vi "EnFlo_Hub.vi"() -> ()   [LabVIEW 2011]
uses:
  Anemometry Sub Vis/Controls/Launch_controls/Open_Calib.ctl
  Anemometry Sub Vis/Controls/Launch_controls/Open_Meas.ctl
  Anemometry Sub Vis/Controls/Launch_controls/Open_Enter_Temp.ctl
  Anemometry Sub Vis/Controls/Launch_controls/Multi_Run_Prog.ctl
  Anemometry Sub Vis/Controls/Launch_controls/EnFlo_arm.ctl
  Anemometry Sub Vis/Controls/Launch_controls/Fast_FID_Valve.ctl
  Anemometry Sub Vis/Controls/Launch_controls/Disp_Setup.ctl
  Anemometry Sub Vis/Controls/Launch_controls/EnFlo_Tun_Setup.ctl
  Anemometry Sub Vis/Controls/Launch_controls/User_Metadata.ctl
  Anemometry Sub Vis/Controls/Launch_controls/Trav_3D_move.ctl
  Anemometry Sub Vis/Controls/Launch_controls/Trav_Space.ctl
  Anemometry Sub Vis/Controls/Launch_controls/Tunnel_speed.ctl
  Anemometry Sub Vis/Controls/Launch_controls/Client_source_control.ctl
  Anemometry Sub Vis/Controls/Launch_controls/Hydrosonic_Manual.ctl
  Anemometry Sub Vis/Controls/Launch_controls/Preference_Panel.ctl
  Anemometry Sub Vis/Controls/Launch_controls/Hot_wire_Calculator.ctl
  Anemometry Sub Vis/Controls/Launch_controls/RW_X_Parker_Config.ctl
  Anemometry Sub Vis/Controls/Launch_controls/LDA_Alignment.ctl
  Anemometry Sub Vis/Controls/Launch_controls/Named_Serial_Comms.ctl
  Anemometry Sub Vis/Controls/Launch_controls/BSA_data_rates.ctl
  Anemometry Sub Vis/Controls/Launch_controls/Serial_Setup.ctl
  Anemometry Sub Vis/Controls/Launch_controls/Post_Process_icon.ctl
  Anemometry Sub Vis/Controls/Launch_controls/Edit_Ascii_file.ctl
  Anemometry Sub Vis/Controls/Launch_controls/Edit_Raw_DF.ctl
  Anemometry Sub Vis/Controls/Launch_controls/Results_file_plotter.ctl
  Anemometry Sub Vis/Controls/Launch_controls/Serial_Port_Names.ctl
  Anemometry Sub Vis/Controls/Launch_controls/Enter_LDA_Setup.ctl
  Anemometry Sub Vis/Controls/Launch_controls/Paul.ctl
  Anemometry Sub Vis/Controls/Launch_controls/Tom.ctl
  Anemometry Sub Vis/Controls/Launch_controls/Scani_Valve.ctl
  Anemometry Sub Vis/Controls/Launch_controls/Edit_sever_Channel.ctl
  Anemometry Sub Vis/Controls/Launch_controls/Day_file_plotter.ctl
  Anemometry Sub Vis/Controls/Launch_controls/Plot_Sever_Data.ctl
  Anemometry Sub Vis/Controls/Launch_controls/Adam_Table.ctl
  Anemometry Sub Vis/Controls/Launch_controls/Active_Channel_Control.ctl
  Anemometry Sub Vis/Controls/Setup.ctl
  Anemometry Sub Vis/Controls/Post_Process.ctl
  Anemometry Sub Vis/Controls/Preference_Mode.ctl
  Anemometry Sub Vis/Gen Trav/Trav_mode.ctl
  Anemometry Sub Vis/Controls/User_Specific_mode.ctl
  Anemometry Sub Vis/File/Setup_Filetype.ctl
  Anemometry Sub Vis/Calibration/Calib_mode.ctl
  Anemometry Sub Vis/Controls/App_Global.ctl
  Anemometry Sub Vis/Globals/Dynamic_call_global.ph.vi
  Anemometry Sub Vis/Globals/Constants_global.vi
  Anemometry Sub Vis/Globals/Preference_global.vi
  Anemometry Sub Vis/Globals/Meas_global.vi
  <vilib>/Platform/browser.llb/Open URL in Default Browser (string).vi
  Anemometry Sub Vis/Globals/Trav_pos_global.vi
  Anemometry Sub Vis/Globals/Qnet_Globals.vi
  Anemometry Sub Vis/Acquisition/PWA/PWAtasksGLOBAL.vi
  Anemometry Sub Vis/Utilities/Email_transfer_global.vi
panel:
  out "List of ADAM channels to view":string[](array[string])
  out "List of ADAM control channels":string[](array[string])
  out "Analogue Dev Name":string="Dev2"
  out "Numeric":i32
  out "Rig Name":string="EnFlo Tunnel"
  out "All Users":path=path "/System Folder/Preferences/LabVIEW (EnFlo specific)/Meas Setups"
  out "Dummy Measurement":bool
  out "Ready to take data?":T1
  out "Local Site Root":path=path "/Lacie_20/paulhayden/Qnet/qnet"
  in  "stop":bool
  in  "Tab Control":T2(tab)
  in  "Tunnel Speed Control":T3
  in  "Traverse Space":T4
  in  "Trav 3D Move":T5 caption="3D Traverse Move"
  in  "User Metadata":T6
  in  "Multi Run Prog":T7
  in  "Enter Temp_Press":T8
  in  "Measurement Prog":T9 caption="Measurement"
  in  "Calibration Prog":T10 caption="Calibration"
  in  "Scani Valve":T11
  in  "LDA Alignment":T12
  in  "Hydrosonic Control":T13
  in  "Fast FID Valve":T14
  in  "Source Control":T15
  in  "Gas Release Setup":T16
  in  "EnFlo Tunnel Setup":T17
  in  "Heater Setup":bool caption="Inlet heater File"
  in  "EnFlo Arm":T18
  in  "Rig_Control":cluster{"Ch Name":string, "Boolean":bool}[](array[cluster])
  in  "ADAM Channels Control":T19 caption="Change Active Channels"
  in  "ADAM Scan Table":T20 caption="Run ADAM Scan Table"
  in  "Edit Server Channel":T21
  in  "Plot Server Channels":T22 caption="Plot Server Data"
  in  "Day Files Plotter":T23 caption="Plot Data From File"
  out "Current Values":cluster{"Ch Name":string, "Numeric":dbl}[](array[cluster])
  in  "Results File Plotter":T24
  in  "Edit Raw Data Files":T25
  in  "Edit ASCII File":T26
  in  "Post Process Raw Data":T27
  in  "LDA Setup":T28
  in  "Port Names":T29
  in  "Serial Setup":T30
  in  "LDA Data Rate":T31
  in  "Named Serial Comms":T32
  in  "RW Trav Setup":T33
  in  "Hot Wire Calc":T34
  in  "Preference Panel":T35
  in  "Tom Lawton t.lawton@surrey.ac.uk":T36 caption="For hardware support"
  in  "Paul Hayden p.hayden@surrey.ac.uk":T37 caption="For software support"
  in  "Online Manual":bool
  out "VI Name":string
  out "Iterations":i32
  # "Or give us a call on Tel: 01483 689545"
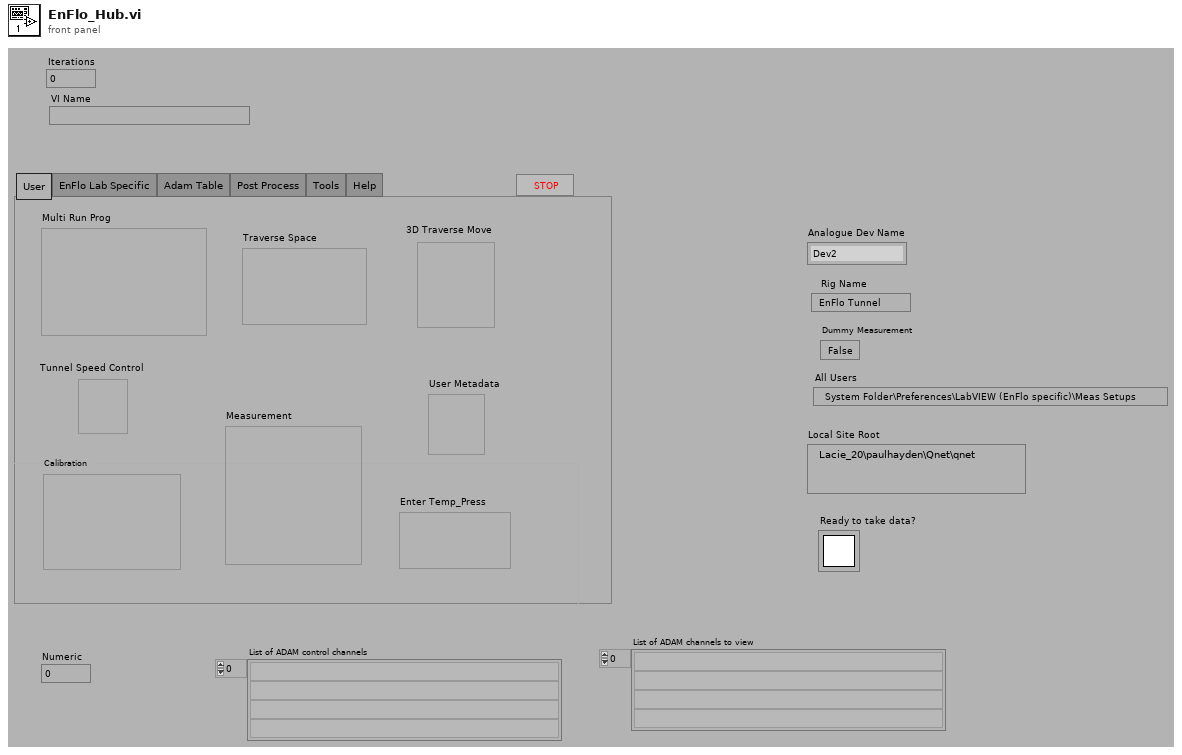
[diagram p1: front panel]
types:
  T1 = typedef "Rendezvous RefNum" = refnum<k1>
  T2 = enum32{"User", "EnFlo Lab Specific", "Adam Table", "Post Process", "Tools", "Help"}
  T3 = typedef "Tunnel_speed.ctl" = bool
  T4 = typedef "Trav_Space.ctl" = bool
  T5 = typedef "Trav_3D_move.ctl" = bool
  T6 = typedef "User_Metadata.ctl" = bool
  T7 = typedef "Multi_Run_Prog.ctl" = bool
  T8 = typedef "Open_Enter_Temp.ctl" = bool
  T9 = typedef "Open_Meas.ctl" = bool
  T10 = typedef "Open_Calib.ctl" = bool
  T11 = typedef "Scani_Valve.ctl" = bool
  T12 = typedef "LDA_Alignment.ctl" = bool
  T13 = typedef "Hydrosonic_Manual.ctl" = bool
  T14 = typedef "Fast_FID_Valve.ctl" = bool
  T15 = typedef "Client_source_control.ctl" = bool
  T16 = typedef "Disp_Setup.ctl" = bool
  T17 = typedef "EnFlo_Tun_Setup.ctl" = bool
  T18 = typedef "EnFlo_arm.ctl" = bool
  T19 = typedef "Active_Channel_Control.ctl" = bool
  T20 = typedef "Adam_Table.ctl" = bool
  T21 = typedef "Edit_sever_Channel.ctl" = bool
  T22 = typedef "Plot_Sever_Data.ctl" = bool
  T23 = typedef "Day_file_plotter.ctl" = bool
  T24 = typedef "Results_file_plotter.ctl" = bool
  T25 = typedef "Edit_Raw_DF.ctl" = bool
  T26 = typedef "Edit_Ascii_file.ctl" = bool
  T27 = typedef "Post_Process_icon.ctl" = bool
  T28 = typedef "Enter_LDA_Setup.ctl" = bool
  T29 = typedef "Serial_Port_Names.ctl" = bool
  T30 = typedef "Serial_Setup.ctl" = bool
  T31 = typedef "BSA_data_rates.ctl" = bool
  T32 = typedef "Named_Serial_Comms.ctl" = bool
  T33 = typedef "RW_X_Parker_Config.ctl" = bool
  T34 = typedef "Hot_wire_Calculator.ctl" = bool
  T35 = typedef "Preference_Panel.ctl" = bool
  T36 = typedef "Tom.ctl" = bool
  T37 = typedef "Paul.ctl" = bool
  T38 = typedef "Post_Process.ctl" = enum16{"Take New Data", "Post Process Raw Data File"}
  T39 = typedef "Setup.ctl" = enum16{"Run Program", "Show Setup", "Save Current Setup", "Setup Front Panel"}
  T40 = enum16{"Get Channel Names", "Get Current Value", "Update Channel Value", "Update Channel Description"}
  T41 = typedef "Preference_Mode.ctl" = enum16{"Load Preferences from file", "Save Preferences to file", "Load, Edit then Save"}
  T42 = typedef "User_Specific_mode.ctl" = enum16{"Check VI only", "Run VI"}
  T43 = typedef "Trav_mode.ctl" = enum16{"Move traverse", "Read traverse position", "Teach Position"}
  T44 = typedef "Setup_Filetype.ctl" = enum16{"Measurement Setups", "Calibration Setups", "General", "Results File Plotter Setups", "Speed Calib Tweaks"}
  T45 = enum16{"Load Command File", "Save Command File", "Check Multi Run Prog", "Check Multi Run Prog With Live Moves", "Run Multi Run Prog"}
  T46 = typedef "Calib_mode.ctl" = enum16{"Show Setup", "Take a New Calibration Point", "Refit Curve", "Setup Front Panel"}
  T47 = typedef "Tunnel_Coordinates.ctl" = enum16{"Work in Tunnel Coordinates", "Work in Model Coordinates"}
  T48 = typedef "App_Global.ctl" = enum16{"Read Global", "Write to Global", "Initialise Array"}
  T49 = typedef "App_Ref_Cluster.ctl" = cluster{"Server IP & Port No":string, "Application reference":refnum<vi>}
  T50 = typedef "Ch_description_ADAM.ctl" = cluster{"Ch Name":string, "Type":T51, "Function":T52, "Ch State":T53, "Calibration type":T54, "A":dbl, "B":dbl, "C":dbl, "D":dbl, "Comments":string, "Address":T55, "String":string, "Duty":u16}
  T51 = typedef "Module_type_ADAM.ctl" = string
  T52 = typedef "Function_ADAM.ctl" = enum16{"Analogue Input", "Digital Input", "Event counter", "Event rate", "Analogue Output", "Digital Output", "Relay Output"}
  T53 = typedef "Channel_State.ctl" = enum16{"On", "Off", "Always On", "Always Off"}
  T54 = typedef "Calib_type_ADAM.ctl" = enum16{"Raw", "Bx + A", "Cx^2 + Bx + A", "Dx^3 + Cx^2 + Bx + A", "In Band", "Hi-Tec Q", "Hi-Tec M_dot", "Text"}
  T55 = typedef "Address.ctl" = cluster{"Main":i32, "Ch.":i32, "Sub":i32, "Port Name":string}
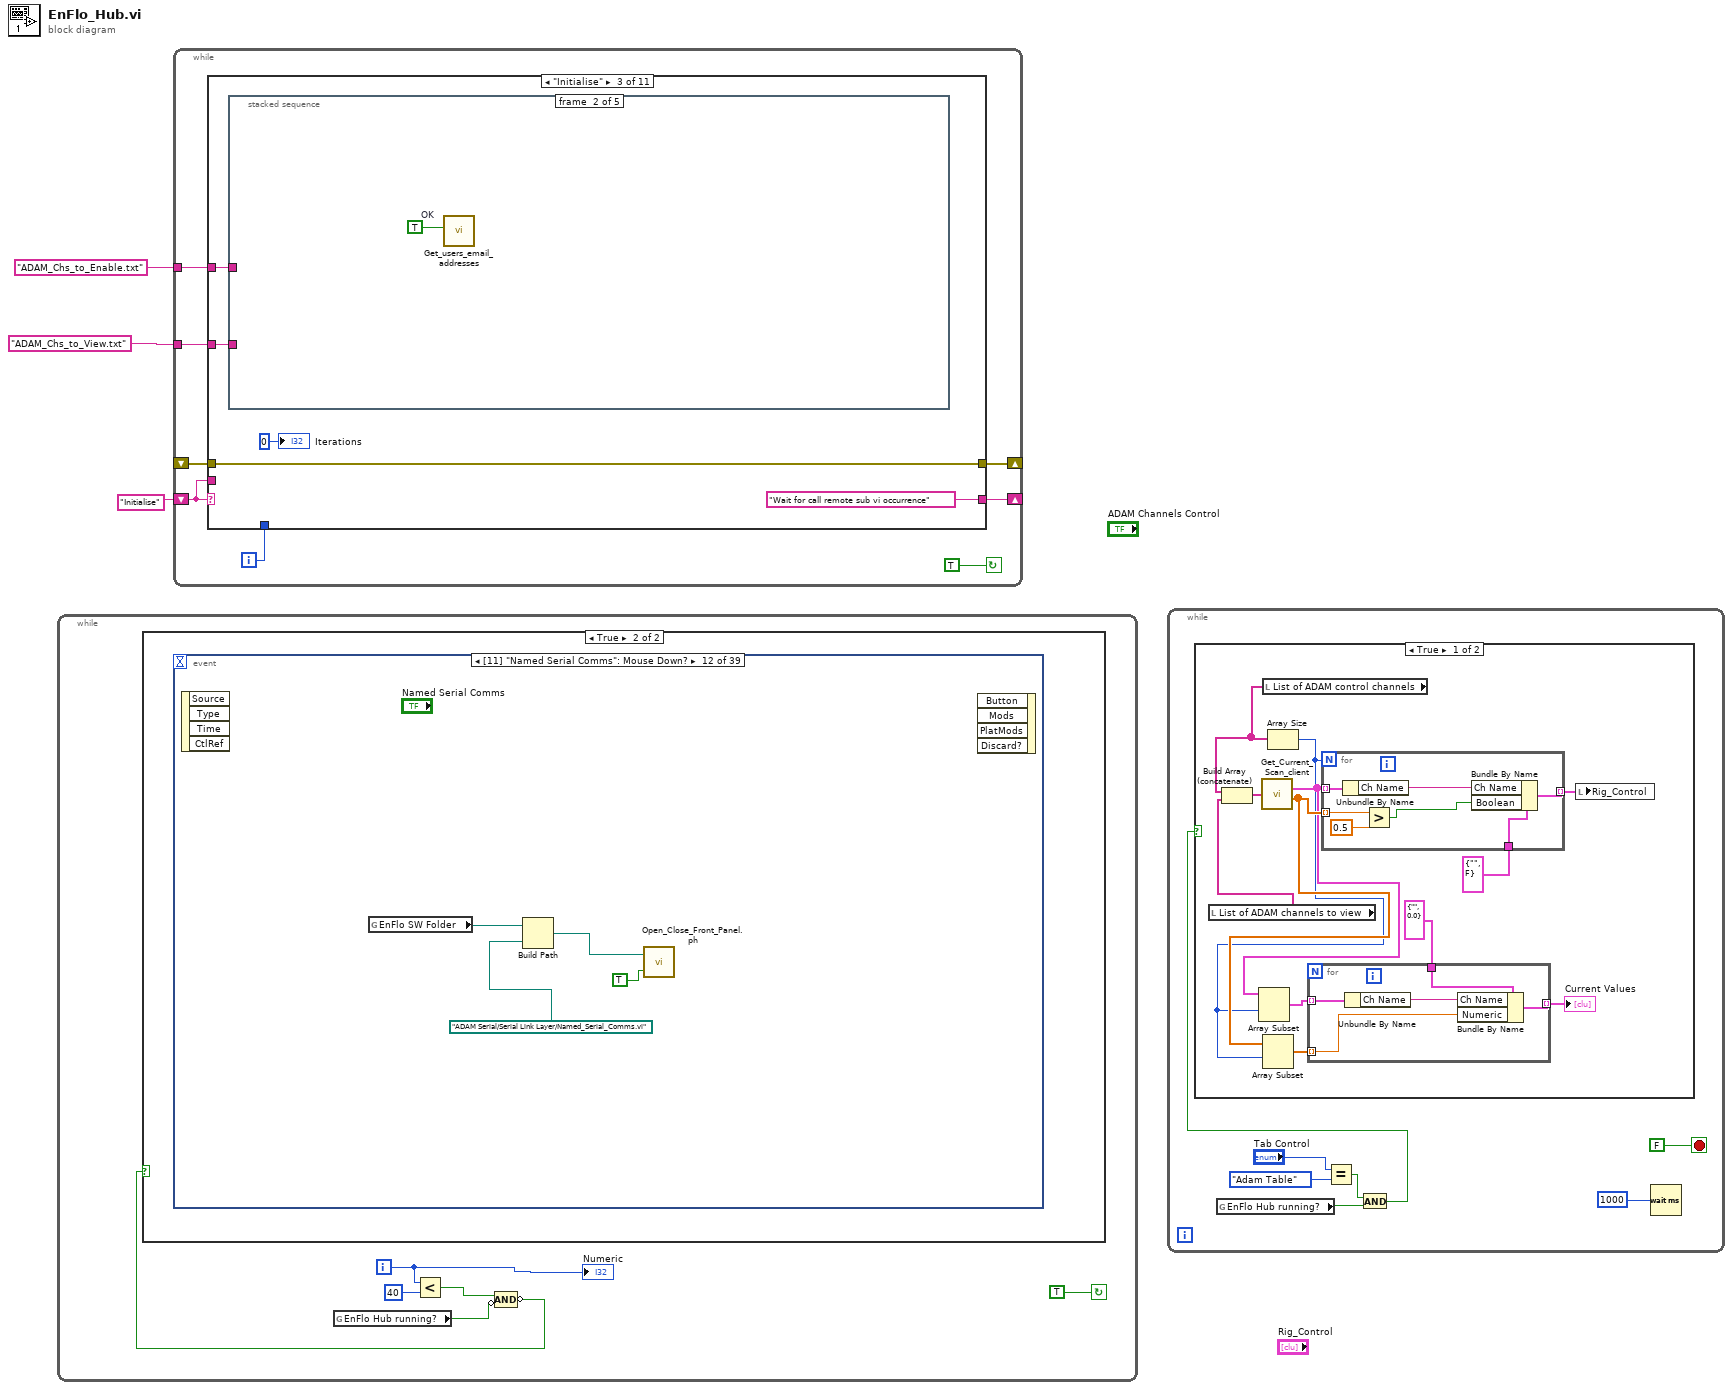
[diagram p0: block diagram]
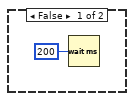
[diagram p3: hidden frame]
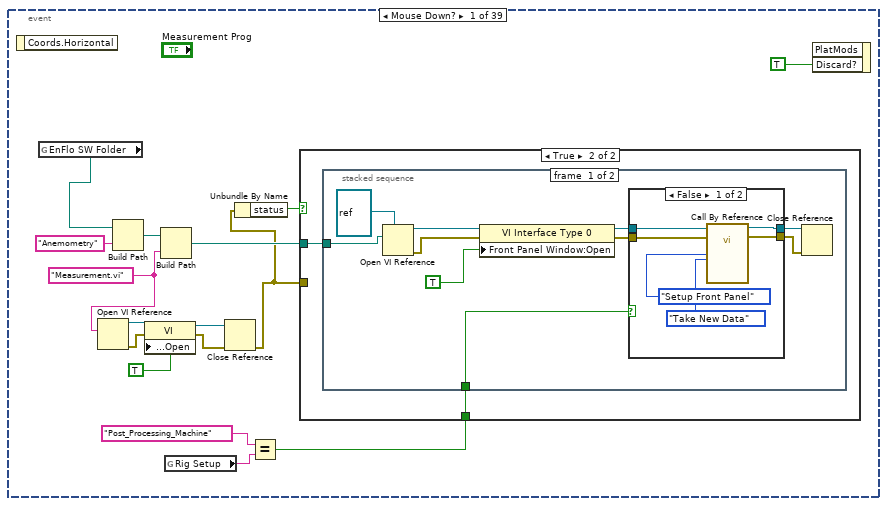
[diagram p4: hidden frame]
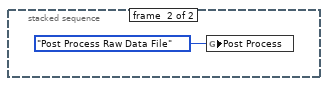
[diagram p7: hidden frame]
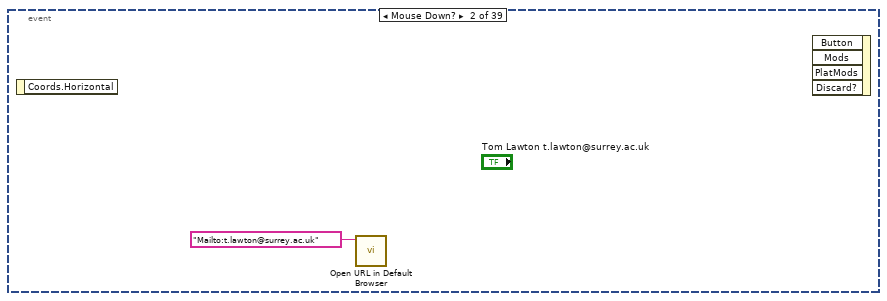
[diagram p8: hidden frame]
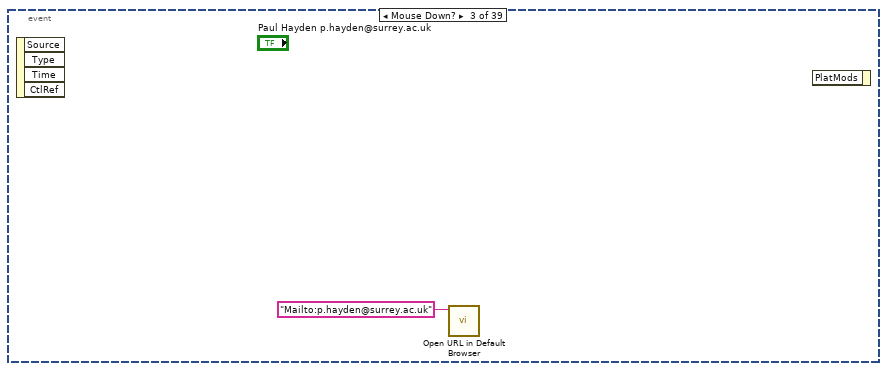
[diagram p9: hidden frame]
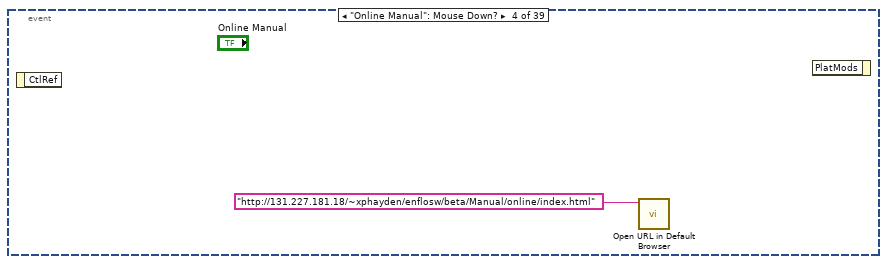
[diagram p10: hidden frame]
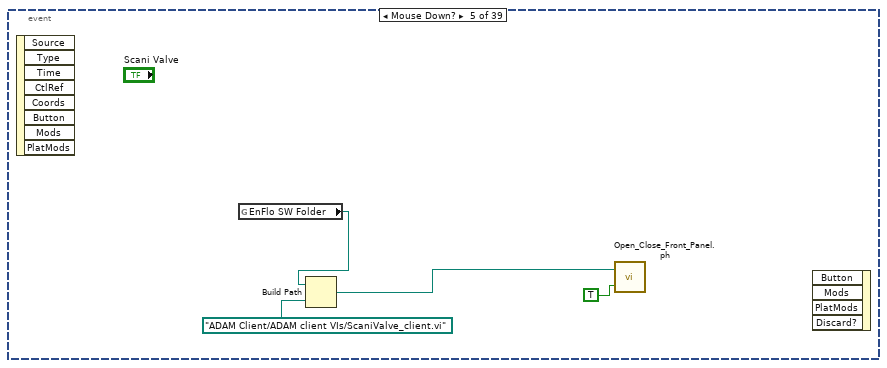
[diagram p11: hidden frame]
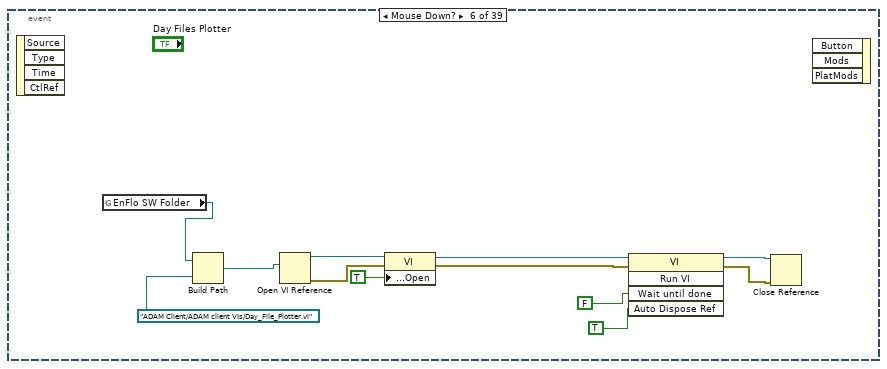
[diagram p12: hidden frame]
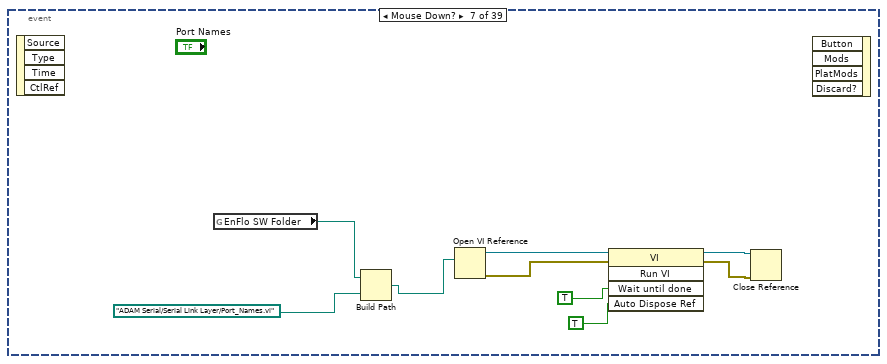
[diagram p13: hidden frame]
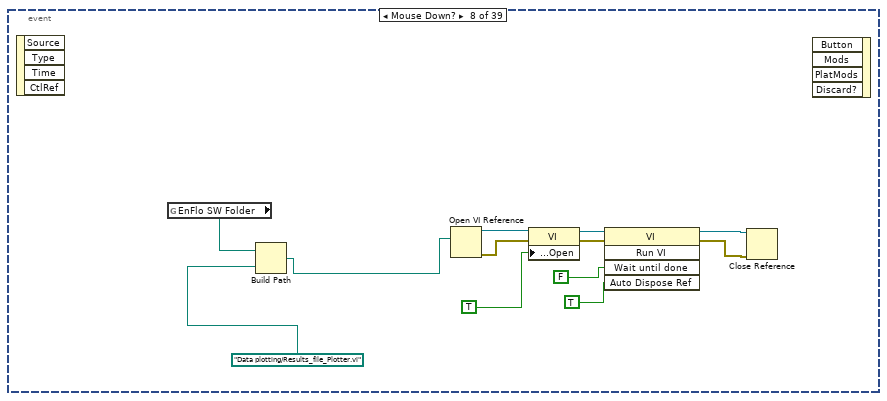
[diagram p14: hidden frame]
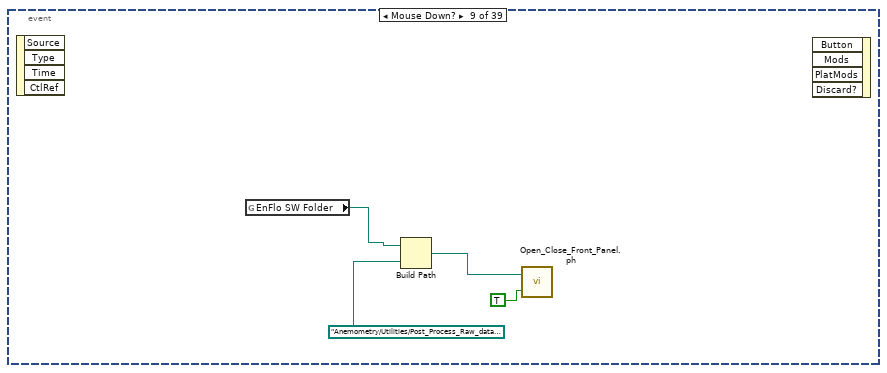
[diagram p15: hidden frame]
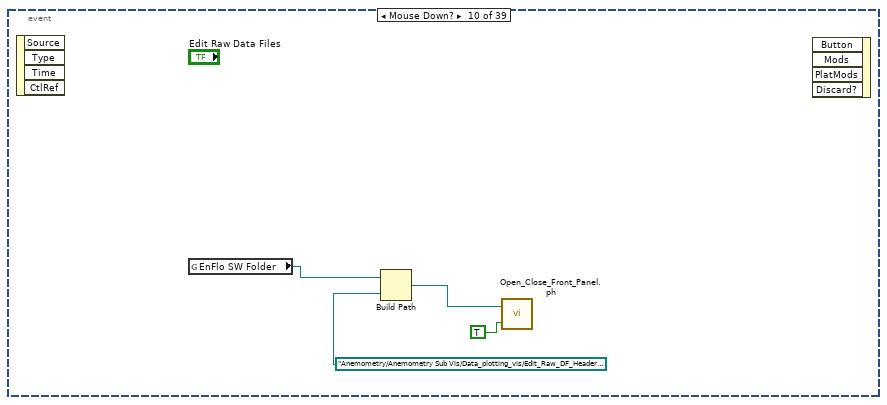
[diagram p16: hidden frame]
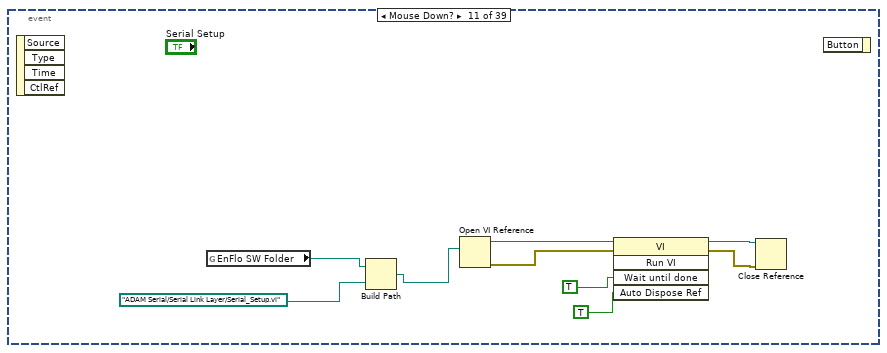
[diagram p17: hidden frame]
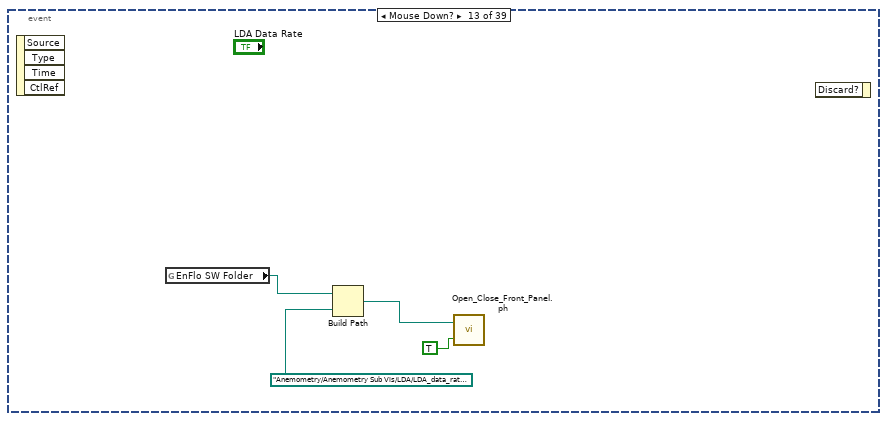
[diagram p18: hidden frame]
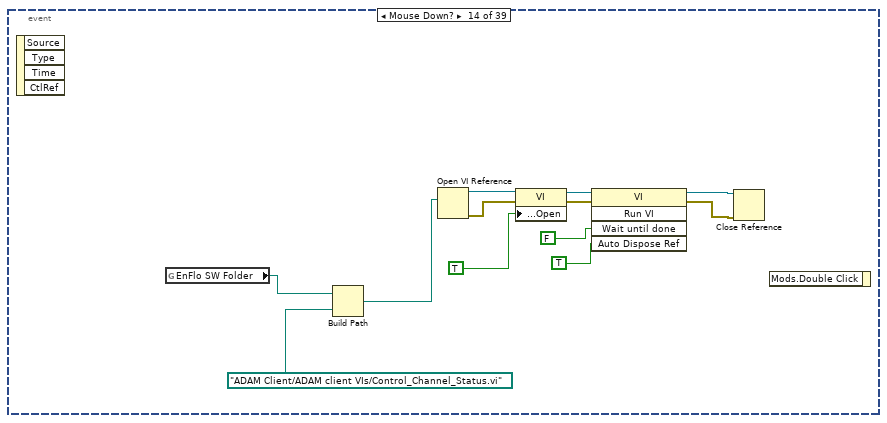
[diagram p19: hidden frame]
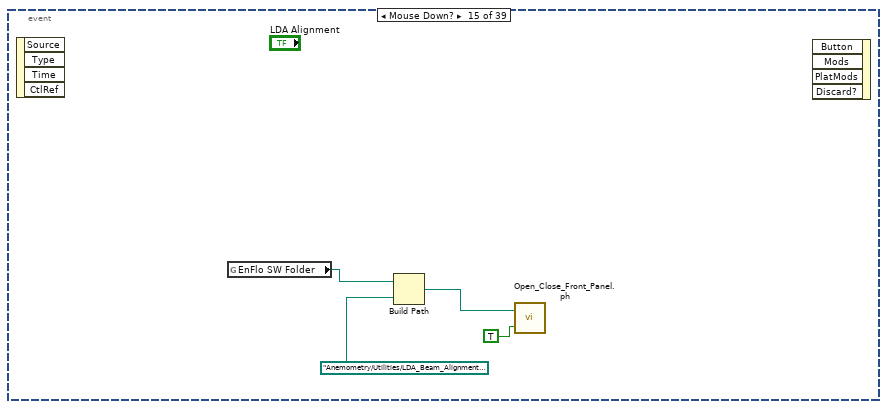
[diagram p20: hidden frame]
diagram:
  n1 = while {
    i -> [w8]
    stop <- TRUE continue-if-true
    n2 = global read "Dynamic_call_global.ph.vi" "EnFlo Hub running?"() -> (w6:bool)
    n3 = Less?(x=w8, y=40) -> (x < y?=w5:bool)
    n4 = Compound Arithmetic op=AND(w5, invert w6) -> (invert w4:bool)
    n5 = case shown="True" w4 {
      frame False {
        n6 = Wait (ms)(milliseconds to wait=u32 200) -> ()  [unwired: 1 out]
      }
      frame True {
        n7 = event shown="[11] \"Named Serial Comms\": Mouse Down?" {
          selector: _ -> [_ _ _ _ _ _ _ _ _ _ _ _ _ _ _ _ _ _ _ _ _ _ _ _ _ _ _ _ _ _ _ _ _ _ _ _ _ _ _]
          dyn-events: _ -> [_ _ _ _ _ _ _ _ _ _ _ _ _ _ _ _ _ _ _ _ _ _ _ _ _ _ _ _ _ _ _ _ _ _ _ _ _ _ _]
          timeout: _ -> [_ _ _ _ _ _ _ _ _ _ _ _ _ _ _ _ _ _ _ _ _ _ _ _ _ _ _ _ _ _ _ _ _ _ _ _ _ _ _]
          event Mouse Down? {
            w19 = "Measurement.vi" ("name or relative path")
            n8 = event-data() -> ()  [unwired: 2 out]
            n9 = global read "Constants_global.vi" "EnFlo SW Folder"() -> (w22:path)
            n10 = Open VI Reference(vi path=w19) -> (vi reference=w18:refnum<vi>, error out=w17:errorcluster)  [unwired: 1 in, 4 out]
            n11 = Build Path(base path=w22, name or relative path="Anemometry") -> (appended path=w25:path)
            n12 = property class="VI"(reference=w18, error in=w17, "Front Panel Window:Open"=TRUE) -> (reference out=w15:refnum<vi>, error out=w16:errorcluster)
            n13 = Build Path(base path=w25, name or relative path=w19) -> (appended path=w23:path)
            n14 = global read "Preference_global.vi" "Rig Setup"() -> (w13:string)
            n15 = Close Reference(reference=w15, error in (no error)=w16) -> (error out=w14:errorcluster)
            n16 = Unbundle By Name(w14) -> ("status"=w24:bool)
            n17 = Equal?(x="Post_Processing_Machine" ("Rig Setup"), y=w13) -> (x = y?=w11:bool)
            n18 = case shown="True" w24 {
              tunnel: w23 -> [_ w28]
              tunnel: w14 -> [_ _]
              tunnel: w11 -> [_ w27]
              frame False {
              }
              frame True {
                n19 = stacked-sequence {
                  tunnel: w28 -> [w38 _]
                  tunnel: w27 -> [w29 _]
                  frame #0 {
                    n20 = Open VI Reference(type specifier VI Refnum (for type only)=refnum<vi> refnum, vi path=w38) -> (vi reference=w36:refnum<vi>, error out=w35:errorcluster)  [unwired: 1 in, 3 out]
                    n21 = property class="VI Interface Type 0"(reference=w36, error in=w35, "Front Panel Window:Open"=TRUE) -> (reference out=w31:refnum<vi>, error out=w30:errorcluster)
                    n22 = case shown="False" w29 {
                      tunnel: [w44 w46] -> w34
                      tunnel: [w43 w45] -> w33
                      tunnel: w31 -> [w42 w46]
                      tunnel: w30 -> [w41 w45]
                      frame False {
                        n23 = call-by-ref "?"(reference=w42, error in=w41, "setup"=Setup."Setup Front Panel", "Post Process"=Post_Process."Take New Data") -> (reference out=w44:refnum<vi>, error out=w43:errorcluster)  [unwired: 16 in, 2 out]
                      }
                      frame True {
                      }
                    }
                    n24 = Close Reference(reference=w34, error in (no error)=w33) -> ()  [unwired: 1 out]
                  }
                  frame #1 {
                    n25 = global write "Meas_global.vi" "Post Process"(Post_Process."Post Process Raw Data File" ("Post Process")) -> ()
                  }
                }
              }
            }
            n26 = event-data("Discard?"=TRUE) -> ()  [unwired: 1 in, 2 out]
          }
          event Mouse Down? {
            n27 = event-data() -> ()  [unwired: 2 out]
            n28 = call-poly <vilib>:"Open URL in Default Browser.vi"("URL"="Mailto:t.lawton@surrey.ac.uk") -> ()  [unwired: 1 in, 6 out]
            n29 = event-data() -> ()  [unwired: 1 in, 5 out]
          }
          event Mouse Down? {
            n30 = event-data() -> ()  [unwired: 5 out]
            n31 = call-poly <vilib>:"Open URL in Default Browser.vi"("URL"="Mailto:p.hayden@surrey.ac.uk") -> ()  [unwired: 1 in, 6 out]
            n32 = event-data() -> ()  [unwired: 1 in, 2 out]
          }
          event "Online Manual": Mouse Down? {
            n33 = event-data() -> ()  [unwired: 2 out]
            n34 = call-poly <vilib>:"Open URL in Default Browser.vi"("URL"="http://131.227.181.18/~xphayden/enflosw/beta/Manual/online/index.html") -> ()  [unwired: 1 in, 6 out]
            n35 = event-data() -> ()  [unwired: 1 in, 2 out]
          }
          event Mouse Down? {
            n36 = event-data() -> ()  [unwired: 9 out]
            n37 = global read "Constants_global.vi" "EnFlo SW Folder"() -> (w51:path)
            n38 = Build Path(base path=w51, name or relative path=path "ADAM Client/ADAM client VIs/ScaniValve_client.vi") -> (appended path=w54:path)
            n39 = call "Open_Close_Front_Panel.ph.vi"("Front Panel Window:Open"=TRUE, "VI path"=w54) -> ()  [unwired: 2 out]
            n40 = event-data() -> ()  [unwired: 1 in, 5 out]
          }
          event Mouse Down? {
            n41 = event-data() -> ()  [unwired: 5 out]
            n42 = global read "Constants_global.vi" "EnFlo SW Folder"() -> (w55:path)
            n43 = Build Path(base path=w55, name or relative path=path "ADAM Client/ADAM client VIs/Day_File_Plotter.vi") -> (appended path=w61:path)
            n44 = Open VI Reference(vi path=w61) -> (vi reference=w62:refnum<vi>, error out=w64:errorcluster)  [unwired: 2 in, 3 out]
            n45 = property class="VI"(reference=w62, error in=w64, "Front Panel Window:Open"=TRUE) -> (reference out=w66:refnum<vi>, error out=w65:errorcluster)
            n46 = invoke class="VI" method="Run VI"(reference=w66, error in=w65, "Wait until done"=FALSE, "Auto Dispose Ref"=TRUE) -> (reference out=w57:refnum<vi>, error out=w58:errorcluster)  [unwired: 1 in, 3 out]
            n47 = Close Reference(reference=w57, error in (no error)=w58) -> ()  [unwired: 1 out]
            n48 = event-data() -> ()  [unwired: 1 in, 4 out]
          }
          event Mouse Down? {
            n49 = event-data() -> ()  [unwired: 5 out]
            n50 = global read "Constants_global.vi" "EnFlo SW Folder"() -> (w67:path)
            n51 = Build Path(base path=w67, name or relative path=path "ADAM Serial/Serial Link Layer/Port_Names.vi") -> (appended path=w69:path)
            n52 = Open VI Reference(vi path=w69) -> (vi reference=w74:refnum<vi>, error out=w75:errorcluster)  [unwired: 1 in, 4 out]
            n53 = invoke class="VI" method="Run VI"(reference=w74, error in=w75, "Wait until done"=TRUE, "Auto Dispose Ref"=TRUE) -> (reference out=w70:refnum<vi>, error out=w71:errorcluster)  [unwired: 1 in, 3 out]
            n54 = Close Reference(reference=w70, error in (no error)=w71) -> ()  [unwired: 1 out]
            n55 = event-data() -> ()  [unwired: 1 in, 5 out]
          }
          event Mouse Down? {
            n56 = event-data() -> ()  [unwired: 5 out]
            n57 = global read "Constants_global.vi" "EnFlo SW Folder"() -> (w76:path)
            n58 = Build Path(base path=w76, name or relative path=path "Data plotting/Results_file_Plotter.vi") -> (appended path=w79:path)
            n59 = Open VI Reference(vi path=w79) -> (vi reference=w81:refnum<vi>, error out=w78:errorcluster)  [unwired: 1 in, 4 out]
            n60 = property class="VI"(reference=w81, error in=w78, "Front Panel Window:Open"=TRUE) -> (reference out=w82:refnum<vi>, error out=w83:errorcluster)
            n61 = invoke class="VI" method="Run VI"(reference=w82, error in=w83, "Wait until done"=FALSE, "Auto Dispose Ref"=TRUE) -> (reference out=w84:refnum<vi>, error out=w85:errorcluster)  [unwired: 1 in, 3 out]
            n62 = Close Reference(reference=w84, error in (no error)=w85) -> ()  [unwired: 1 out]
            n63 = event-data() -> ()  [unwired: 1 in, 5 out]
          }
          event Mouse Down? {
            n64 = event-data() -> ()  [unwired: 5 out]
            n65 = global read "Constants_global.vi" "EnFlo SW Folder"() -> (w88:path)
            n66 = Build Path(base path=w88, name or relative path=path "Anemometry/Utilities/Post_Process_Raw_data.vi") -> (appended path=w90:path)
            n67 = call "Open_Close_Front_Panel.ph.vi"("Front Panel Window:Open"=TRUE, "VI path"=w90) -> ()  [unwired: 2 out]
            n68 = event-data() -> ()  [unwired: 1 in, 5 out]
          }
          event Mouse Down? {
            n69 = event-data() -> ()  [unwired: 5 out]
            n70 = global read "Constants_global.vi" "EnFlo SW Folder"() -> (w92:path)
            n71 = Build Path(base path=w92, name or relative path=path "Anemometry/Anemometry Sub Vis/Data_plotting_vis/Edit_Raw_DF_Header.vi") -> (appended path=w94:path)
            n72 = call "Open_Close_Front_Panel.ph.vi"("Front Panel Window:Open"=TRUE, "VI path"=w94) -> ()  [unwired: 2 out]
            n73 = event-data() -> ()  [unwired: 1 in, 5 out]
          }
          event Mouse Down? {
            n74 = event-data() -> ()  [unwired: 5 out]
            n75 = global read "Constants_global.vi" "EnFlo SW Folder"() -> (w96:path)
            n76 = Build Path(base path=w96, name or relative path=path "ADAM Serial/Serial Link Layer/Serial_Setup.vi") -> (appended path=w98:path)
            n77 = Open VI Reference(vi path=w98) -> (vi reference=w103:refnum<vi>, error out=w104:errorcluster)  [unwired: 1 in, 4 out]
            n78 = invoke class="VI" method="Run VI"(reference=w103, error in=w104, "Wait until done"=TRUE, "Auto Dispose Ref"=TRUE) -> (reference out=w99:refnum<vi>, error out=w100:errorcluster)  [unwired: 1 in, 3 out]
            n79 = Close Reference(reference=w99, error in (no error)=w100) -> ()  [unwired: 1 out]
            n80 = event-data() -> ()  [unwired: 1 in, 2 out]
          }
          event Mouse Down? {
            n81 = event-data() -> ()  [unwired: 5 out]
            n82 = global read "Constants_global.vi" "EnFlo SW Folder"() -> (w106:path)
            n83 = Build Path(base path=w106, name or relative path=path "ADAM Serial/Serial Link Layer/Named_Serial_Comms.vi") -> (appended path=w108:path)
            n84 = call "Open_Close_Front_Panel.ph.vi"("Front Panel Window:Open"=TRUE, "VI path"=w108) -> ()  [unwired: 2 out]
            n85 = event-data() -> ()  [unwired: 1 in, 5 out]
          }
          event Mouse Down? {
            n86 = event-data() -> ()  [unwired: 5 out]
            n87 = global read "Constants_global.vi" "EnFlo SW Folder"() -> (w109:path)
            n88 = Build Path(base path=w109, name or relative path=path "Anemometry/Anemometry Sub Vis/LDA/LDA_data_rate.vi") -> (appended path=w111:path)
            n89 = call "Open_Close_Front_Panel.ph.vi"("Front Panel Window:Open"=TRUE, "VI path"=w111) -> ()  [unwired: 2 out]
            n90 = event-data() -> ()  [unwired: 1 in, 2 out]
          }
          event Mouse Down? {
            n91 = event-data() -> ()  [unwired: 5 out]
            n92 = global read "Constants_global.vi" "EnFlo SW Folder"() -> (w123:path)
            n93 = Build Path(base path=w123, name or relative path=path "ADAM Client/ADAM client VIs/Control_Channel_Status.vi") -> (appended path=w113:path)
            n94 = Open VI Reference(vi path=w113) -> (vi reference=w116:refnum<vi>, error out=w114:errorcluster)  [unwired: 1 in, 4 out]
            n95 = property class="VI"(reference=w116, error in=w114, "Front Panel Window:Open"=TRUE) -> (reference out=w117:refnum<vi>, error out=w118:errorcluster)
            n96 = invoke class="VI" method="Run VI"(reference=w117, error in=w118, "Wait until done"=FALSE, "Auto Dispose Ref"=TRUE) -> (reference out=w119:refnum<vi>, error out=w120:errorcluster)  [unwired: 1 in, 3 out]
            n97 = Close Reference(reference=w119, error in (no error)=w120) -> ()  [unwired: 1 out]
            n98 = event-data() -> ()  [unwired: 1 in, 2 out]
          }
          event Mouse Down? {
            n99 = event-data() -> ()  [unwired: 5 out]
            n100 = global read "Constants_global.vi" "EnFlo SW Folder"() -> (w125:path)
            n101 = Build Path(base path=w125, name or relative path=path "Anemometry/Utilities/LDA_Beam_Alignment.vi") -> (appended path=w127:path)
            n102 = call "Open_Close_Front_Panel.ph.vi"("Front Panel Window:Open"=TRUE, "VI path"=w127) -> ()  [unwired: 2 out]
            n103 = event-data() -> ()  [unwired: 1 in, 5 out]
          }
          event Mouse Down? {
            w130 = FALSE  # Wait until done
            n104 = event-data() -> ()  [unwired: 5 out]
            n105 = call "Run_Enter_Temp.vi"("Wait until done"=w130) -> ()  [unwired: 1 out]
            n106 = event-data("Discard?"=TRUE) -> ()  [unwired: 1 in, 4 out]
          }
          event Mouse Down? {
            n107 = event-data() -> ()  [unwired: 5 out]
            n108 = global read "Constants_global.vi" "EnFlo SW Folder"() -> (w131:path)
            n109 = Build Path(base path=w131, name or relative path=path "Anemometry/Utilities/Edit_ASCI_file.vi") -> (appended path=w134:path)
            n110 = call "Open_Close_Front_Panel.ph.vi"("Front Panel Window:Open"=TRUE, "VI path"=w134) -> ()  [unwired: 2 out]
            n111 = event-data() -> ()  [unwired: 1 in, 5 out]
          }
          event "Heater Setup": Mouse Down? {
            n112 = event-data() -> ()  [unwired: 5 out]
            n113 = global read "Constants_global.vi" "EnFlo SW Folder"() -> (w135:path)
            n114 = Build Path(base path=w135, name or relative path=path "Anemometry/Utilities/Create_Heater_Setpoints_File.vi") -> (appended path=w138:path)
            n115 = call "Open_Close_Front_Panel.ph.vi"("Front Panel Window:Open"=TRUE, "VI path"=w138) -> ()  [unwired: 2 out]
            n116 = event-data() -> ()  [unwired: 1 in, 5 out]
          }
          event Mouse Down? {
            n117 = event-data() -> ()  [unwired: 5 out]
            n118 = global read "Constants_global.vi" "EnFlo SW Folder"() -> (w139:path)
            n119 = Build Path(base path=w139, name or relative path=path "ADAM Client/Sub VIs/Gas_Release_Control.vi") -> (appended path=w142:path)
            n120 = call "Open_Close_Front_Panel.ph.vi"("Front Panel Window:Open"=TRUE, "VI path"=w142) -> ()  [unwired: 2 out]
            n121 = event-data() -> ()  [unwired: 1 in, 5 out]
          }
          event Mouse Down? {
            n122 = event-data() -> ()  [unwired: 5 out]
            n123 = global read "Constants_global.vi" "EnFlo SW Folder"() -> (w143:path)
            n124 = Build Path(base path=w143, name or relative path=path "ADAM Client/ADAM client VIs/Edit_Server_Channel.vi") -> (appended path=w153:path)
            n125 = Open VI Reference(type specifier VI Refnum (for type only)=refnum<vi> refnum, vi path=w153) -> (vi reference=w146:refnum<vi>, error out=w147:errorcluster)  [unwired: 1 in, 3 out]
            n126 = property class="VI Interface Type 1"(reference=w146, error in=w147, "Front Panel Window:Open"=TRUE) -> (reference out=w149:refnum<vi>, error out=w150:errorcluster)
            n127 = call-by-ref "?"(reference=w149, error in=w150, "Mode"=T40."Get Channel Names") -> (reference out=w151:refnum<vi>, error out=w152:errorcluster)  [unwired: 5 in]
            n128 = Close Reference(reference=w151, error in (no error)=w152) -> ()  [unwired: 1 out]
            n129 = event-data() -> ()  [unwired: 1 in, 5 out]
          }
          event Mouse Down? {
            n130 = event-data() -> ()  [unwired: 5 out]
            n131 = global read "Constants_global.vi" "EnFlo SW Folder"() -> (w155:path)
            n132 = Build Path(base path=w155, name or relative path=path "ADAM Client/ADAM client VIs/Set_Tunnel_Speed.vi") -> (appended path=w158:path)
            n133 = call "Open_Close_Front_Panel.ph.vi"("Front Panel Window:Open"=TRUE, "VI path"=w158) -> ()  [unwired: 2 out]
            n134 = event-data() -> ()  [unwired: 1 in, 5 out]
          }
          event Mouse Down? {
            n135 = event-data() -> ()  [unwired: 5 out]
            n136 = global read "Constants_global.vi" "EnFlo SW Folder"() -> (w159:path)
            n137 = Build Path(base path=w159, name or relative path=path "ADAM Client/ADAM client VIs/Plot_Server_Data.vi") -> (appended path=w162:path)
            n138 = Open VI Reference(vi path=w162) -> (vi reference=w164:refnum<vi>, error out=w161:errorcluster)  [unwired: 1 in, 4 out]
            n139 = property class="VI"(reference=w164, error in=w161, "Front Panel Window:Open"=TRUE) -> (reference out=w165:refnum<vi>, error out=w166:errorcluster)
            n140 = invoke class="VI" method="Run VI"(reference=w165, error in=w166, "Wait until done"=FALSE, "Auto Dispose Ref"=TRUE) -> (reference out=w167:refnum<vi>, error out=w168:errorcluster)  [unwired: 1 in, 3 out]
            n141 = Close Reference(reference=w167, error in (no error)=w168) -> ()  [unwired: 1 out]
            n142 = event-data() -> ()  [unwired: 1 in, 5 out]
          }
          event Mouse Down? {
            n143 = event-data() -> ()  [unwired: 5 out]
            n144 = Two Button Dialog(message="Are you sure that you want to Run the ADAM Scan table on this machine?", 1:"Run" ("F button name (\"Cancel\")"), 2:"Cancel" ("T button name (\"OK\")")) -> (T button?=w172:bool)
            n145 = case shown="False" w172 {
              frame False {
                n146 = global read "Constants_global.vi" "EnFlo SW Folder"() -> (w175:path)
                n147 = Build Path(base path=w175, name or relative path=path "ADAM Server/ADAM_scan_table.vi") -> (appended path=w178:path)
                n148 = Open VI Reference(vi path=w178) -> (vi reference=w180:refnum<vi>, error out=w177:errorcluster)  [unwired: 1 in, 4 out]
                n149 = property class="VI"(reference=w180, error in=w177, "Front Panel Window:Open"=TRUE) -> (reference out=w181:refnum<vi>, error out=w182:errorcluster)
                n150 = invoke class="VI" method="Run VI"(reference=w181, error in=w182, "Wait until done"=FALSE, "Auto Dispose Ref"=TRUE) -> (reference out=w183:refnum<vi>, error out=w184:errorcluster)  [unwired: 1 in, 3 out]
                n151 = Close Reference(reference=w183, error in (no error)=w184) -> ()  [unwired: 1 out]
              }
              frame True {
              }
            }
            n152 = event-data() -> ()  [unwired: 1 in, 2 out]
          }
          event Mouse Down? {
            n153 = event-data() -> ()  [unwired: 5 out]
            n154 = global read "Constants_global.vi" "EnFlo SW Folder"() -> (w189:path)
            n155 = Build Path(base path=w189, name or relative path=path "ADAM Serial/Instrument drivers/Traverses/~subVIs/Read_Write_Trav_Config.vi") -> (appended path=w190:path)
            n156 = Build Path(base path=w189, name or relative path=path "ADAM Serial/Instrument drivers/Traverses/~subVIs/DriveConfigGlobal.vi") -> (appended path=w191:path)
            n157 = flat-sequence {
              tunnel: w191 -> [w192]
              tunnel: w190 -> [w194]
              frame #0 {
                n158 = call "Open_Close_Front_Panel.ph.vi"("Front Panel Window:Open"=TRUE, "VI path"=w192) -> ()  [unwired: 2 out]
              }
              frame #1 {
                n159 = call "Open_Close_Front_Panel.ph.vi"("Front Panel Window:Open"=TRUE, "VI path"=w194) -> ()  [unwired: 2 out]
              }
            }
            n160 = event-data() -> ()  [unwired: 1 in, 5 out]
          }
          event Mouse Down? {
            n161 = event-data() -> ()  [unwired: 5 out]
            n162 = global read "Constants_global.vi" "EnFlo SW Folder"() -> (w196:path)
            n163 = Build Path(base path=w196, name or relative path=path "Anemometry/Utilities/Hot_wire_Calculator.vi") -> (appended path=w199:path)
            n164 = call "Open_Close_Front_Panel.ph.vi"("Front Panel Window:Open"=TRUE, "VI path"=w199) -> ()  [unwired: 2 out]
            n165 = event-data() -> ()  [unwired: 1 in, 5 out]
          }
          event Mouse Down? {
            n166 = event-data() -> ()  [unwired: 5 out]
            n167 = global read "Constants_global.vi" "EnFlo SW Folder"() -> (w200:path)
            n168 = Build Path(base path=w200, name or relative path=path "Anemometry/Utilities/Hydrosonic_Manual.vi") -> (appended path=w203:path)
            n169 = call "Open_Close_Front_Panel.ph.vi"("Front Panel Window:Open"=TRUE, "VI path"=w203) -> ()  [unwired: 2 out]
            n170 = event-data() -> ()  [unwired: 1 in, 5 out]
          }
          event Mouse Down? {
            n171 = event-data() -> ()  [unwired: 5 out]
            n172 = global read "Constants_global.vi" "EnFlo SW Folder"() -> (w204:path)
            n173 = Build Path(base path=w204, name or relative path=path "ADAM Client/ADAM client VIs/Fast_FID_Valve_Control.vi") -> (appended path=w207:path)
            n174 = call "Open_Close_Front_Panel.ph.vi"("Front Panel Window:Open"=TRUE, "VI path"=w207) -> ()  [unwired: 2 out]
            n175 = event-data() -> ()  [unwired: 1 in, 5 out]
          }
          event Mouse Down? {
            n176 = event-data() -> ()  [unwired: 5 out]
            n177 = global read "Constants_global.vi" "EnFlo SW Folder"() -> (w208:path)
            n178 = Build Path(base path=w208, name or relative path=path "Anemometry/Utilities/Preference_Panel.vi") -> (appended path=w217:path)
            n179 = Open VI Reference(type specifier VI Refnum (for type only)=refnum<vi> refnum, vi path=w217) -> (vi reference=w210:refnum<vi>, error out=w211:errorcluster)  [unwired: 1 in, 3 out]
            n180 = property class="VI Interface Type 2"(reference=w210, error in=w211, "Front Panel Window:Open"=TRUE) -> (reference out=w213:refnum<vi>, error out=w214:errorcluster)
            n181 = call-by-ref "?"(reference=w213, error in=w214, "Mode"=Preference_Mode."Load, Edit then Save") -> (reference out=w215:refnum<vi>, error out=w216:errorcluster)
            n182 = Close Reference(reference=w215, error in (no error)=w216) -> ()  [unwired: 1 out]
            n183 = event-data("Discard?"=TRUE) -> ()  [unwired: 1 in, 4 out]
          }
          event Mouse Down? {
            n184 = event-data() -> ()  [unwired: 5 out]
            n185 = global read "Constants_global.vi" "EnFlo SW Folder"() -> (w224:path)
            n186 = Build Path(base path=w224, name or relative path=path "ADAM Client/Sub VIs/Gas_Setup.vi") -> (appended path=w231:path)
            n187 = Open VI Reference(type specifier VI Refnum (for type only)=refnum<vi> refnum, vi path=w231) -> (vi reference=w227:refnum<vi>, error out=w228:errorcluster)  [unwired: 1 in, 3 out]
            n188 = property class="VI Interface Type 3"(reference=w227, error in=w228, "Front Panel Window:Open"=TRUE) -> (reference out=w232:refnum<vi>, error out=w230:errorcluster)
            n189 = call-by-ref "?"(reference=w232, error in=w230) -> (reference out=w222:refnum<vi>, error out=w221:errorcluster)  [unwired: 9 in]
            n190 = Close Reference(reference=w222, error in (no error)=w221) -> ()  [unwired: 1 out]
            n191 = event-data("Discard?"=TRUE) -> ()  [unwired: 1 in, 4 out]
          }
          event Mouse Down? {
            n192 = event-data() -> ()  [unwired: 5 out]
            n193 = global read "Constants_global.vi" "EnFlo SW Folder"() -> (w236:path)
            n194 = Build Path(base path=w236, name or relative path=path "ADAM Client/Sub VIs/User_Metadata.vi") -> (appended path=w243:path)
            n195 = Open VI Reference(type specifier VI Refnum (for type only)=refnum<vi> refnum, vi path=w243) -> (vi reference=w239:refnum<vi>, error out=w240:errorcluster)  [unwired: 1 in, 3 out]
            n196 = property class="VI Interface Type 3"(reference=w239, error in=w240, "Front Panel Window:Open"=TRUE) -> (reference out=w244:refnum<vi>, error out=w242:errorcluster)
            n197 = call-by-ref "?"(reference=w244, error in=w242) -> (reference out=w234:refnum<vi>, error out=w233:errorcluster)  [unwired: 9 in]
            n198 = Close Reference(reference=w234, error in (no error)=w233) -> ()  [unwired: 1 out]
            n199 = event-data("Discard?"=TRUE) -> ()  [unwired: 1 in, 4 out]
          }
          event Mouse Down? {
            n200 = event-data() -> ()  [unwired: 5 out]
            n201 = global read "Constants_global.vi" "EnFlo SW Folder"() -> (w250:path)
            n202 = Build Path(base path=w250, name or relative path=path "ADAM Client/Sub VIs/EnFlo_Tunnel_Setup.vi") -> (appended path=w253:path)
            n203 = Open VI Reference(type specifier VI Refnum (for type only)=refnum<vi> refnum, vi path=w253) -> (vi reference=w247:refnum<vi>, error out=w246:errorcluster)  [unwired: 1 in, 3 out]
            n204 = call-by-ref "?"(reference=w247, error in=w246) -> (reference out=w249:refnum<vi>, error out=w248:errorcluster)  [unwired: 9 in]
            n205 = Close Reference(reference=w249, error in (no error)=w248) -> ()  [unwired: 1 out]
            n206 = event-data("Discard?"=TRUE) -> ()  [unwired: 1 in, 4 out]
          }
          event Mouse Down? {
            w264 = TRUE  # Show Panel?
            n207 = event-data() -> ()  [unwired: 5 out]
            n208 = global read "Constants_global.vi" "EnFlo SW Folder"() -> (w259:path)
            n209 = Build Path(base path=w259, name or relative path=path "Anemometry/Anemometry Sub Vis/Gen Trav/Traverse_Space.vi") -> (appended path=w262:path)
            n210 = global read "Trav_pos_global.vi" "Default Traverse Setup"() -> (w254:string)
            n211 = Open VI Reference(type specifier VI Refnum (for type only)=refnum<vi> refnum, vi path=w262) -> (vi reference=w263:refnum<vi>, error out=w255:errorcluster)  [unwired: 1 in, 3 out]
            n212 = call-by-ref "?"(reference=w263, error in=w255, "Show Panel?"=w264, "Traverse Setup"=w254) -> (reference out=w257:refnum<vi>, error out=w256:errorcluster)  [unwired: 8 in, 1 out]
            n213 = Close Reference(reference=w257, error in (no error)=w256) -> ()  [unwired: 1 out]
            n214 = event-data("Discard?"=TRUE) -> ()  [unwired: 1 in, 4 out]
          }
          event Mouse Down? {
            n215 = event-data() -> ()  [unwired: 5 out]
            n216 = global read "Constants_global.vi" "EnFlo SW Folder"() -> (w266:path)
            n217 = Build Path(base path=w266, name or relative path=path "Anemometry/Anemometry Sub Vis/Traverse vi's/EnFlo Tunnel specific/Check_EnFlo_Arm.vi") -> (appended path=w268:path)
            n218 = call "Open_Close_Front_Panel.ph.vi"("Front Panel Window:Open"=TRUE, "VI path"=w268) -> ()  [unwired: 2 out]
            n219 = event-data() -> ()  [unwired: 1 in, 2 out]
          }
          event Mouse Down? {
            n220 = event-data() -> ()  [unwired: 5 out]
            n221 = global read "Constants_global.vi" "EnFlo SW Folder"() -> (w276:path)
            n222 = Build Path(base path=w276, name or relative path=path "Anemometry/Anemometry Sub Vis/Gen Trav/3D_Traverse_move.vi") -> (appended path=w273:path)
            n223 = Strip Path(path=w273) -> (name=w272:string)  [unwired: 1 out]
            n224 = Open VI Reference(vi path=w272) -> (vi reference=w274:refnum<vi>, error out=w275:errorcluster)  [unwired: 1 in, 4 out]
            n225 = property class="VI"(reference=w274, error in=w275) -> (reference out=w270:refnum<vi>, error out=w269:errorcluster, "Front Panel Window:Open"=w271:bool)
            n226 = case shown="False" w271 {
              tunnel: w273 -> [w278 _]
              tunnel: w270 -> [_ w295]
              tunnel: w269 -> [_ w294]
              frame False {
                n227 = global read "Trav_pos_global.vi" "Work in Tunnel Coordinates?"() -> (w288:T47)
                n228 = global read "Trav_pos_global.vi" "Default Traverse Setup"() -> (w286:string)
                n229 = Open VI Reference(type specifier VI Refnum (for type only)=refnum<vi> refnum, vi path=w278) -> (vi reference=w282:refnum<vi>, error out=w283:errorcluster)  [unwired: 1 in, 3 out]
                n230 = property class="VI Interface Type 4"(reference=w282, error in=w283, "Front Panel Window:Open"=TRUE) -> (reference out=w279:refnum<vi>, error out=w280:errorcluster)
                n231 = call-by-ref "?"(reference=w279, error in=w280, "Mode"=Trav_mode."Read traverse position", "Work in Tunnel Coordinates"=w288, "Simulate/Run"=User_Specific_mode."Run VI", "Traverse name"=w286) -> (reference out=w284:refnum<vi>, error out=w285:errorcluster)  [unwired: 9 in, 3 out]
                n232 = Close Reference(reference=w284, error in (no error)=w285) -> ()  [unwired: 1 out]
              }
              frame True {
                n233 = property class="VI"(reference=w295, error in=w294, "Front Panel Window:Open"=TRUE) -> (reference out=w293:refnum<vi>, error out=w292:errorcluster)
                n234 = Close Reference(reference=w293, error in (no error)=w292) -> ()  [unwired: 1 out]
              }
            }
            n235 = event-data() -> ()  [unwired: 1 in, 5 out]
          }
          event Mouse Down? {
            n236 = event-data() -> ()  [unwired: 5 out]
            n237 = Open VI Reference(vi path="Multi_Run_Prog.vi") -> (vi reference=w301:refnum<vi>, error out=w300:errorcluster)  [unwired: 1 in, 4 out]
            n238 = property class="VI"(reference=w301, error in=w300, "Front Panel Window:Open"=TRUE) -> (reference out=w298:refnum<vi>, error out=w299:errorcluster)
            n239 = Close Reference(reference=w298, error in (no error)=w299) -> (error out=w296:errorcluster)
            n240 = Unbundle By Name(w296) -> ("status"=w303:bool)
            n241 = case shown="True" w303 {
              frame False {
              }
              frame True {
                n242 = global read "Constants_global.vi" "EnFlo SW Folder"() -> (w311:path)
                n243 = call "Setup_Filepath.vi"("Setup File Type"=Setup_Filetype."General", "Filename in"="Multi_Run_Filename.txt" ("name or relative path")) -> ("Filename Out"=w304:path)  [unwired: 1 out]
                n244 = Build Path(base path=w311, name or relative path=path "Anemometry/Multi_Run_Prog.vi") -> (appended path=w310:path)
                n245 = call "Read_File_Simple.vi"("Filename"=w304) -> ("string"=w309:string)  [unwired: 2 in, 7 out]
                n246 = String To Path(string=w309) -> (path=w307:path)
                n247 = call "Does_file_exist_(simple).vi"("Pathname"=w307) -> ("exists?"=w308:bool)
                n248 = case shown="False" w308 {
                  tunnel: w310 -> [w313 w325]
                  tunnel: w307 -> [_ w322]
                  frame False {
                    n249 = call "Open_Close_Front_Panel.ph.vi"("Front Panel Window:Open"=TRUE, "VI path"=w313) -> ()  [unwired: 2 out]
                  }
                  frame True {
                    n250 = Open VI Reference(type specifier VI Refnum (for type only)=refnum<vi> refnum, vi path=w325) -> (vi reference=w321:refnum<vi>, error out=w320:errorcluster)  [unwired: 1 in, 3 out]
                    n251 = property class="VI Interface Type 5"(reference=w321, error in=w320, "Front Panel Window:Open"=TRUE) -> (reference out=w318:refnum<vi>, error out=w319:errorcluster)
                    n252 = call-by-ref "?"(reference=w318, error in=w319, "Command filename"=w322, "Setup mode"=T45."Load Command File") -> (reference out=w317:refnum<vi>, error out=w316:errorcluster)  [unwired: 18 in]
                    n253 = Close Reference(reference=w317, error in (no error)=w316) -> ()  [unwired: 1 out]
                  }
                }
              }
            }
            n254 = event-data() -> ()  [unwired: 1 in, 5 out]
          }
          event Mouse Down? {
            w327 = "Calibration.vi" ("name or relative path")
            n255 = event-data() -> ()  [unwired: 5 out]
            n256 = global read "Constants_global.vi" "EnFlo SW Folder"() -> (w333:path)
            n257 = Open VI Reference(vi path=w327) -> (vi reference=w331:refnum<vi>, error out=w330:errorcluster)  [unwired: 1 in, 4 out]
            n258 = Build Path(base path=w333, name or relative path="Anemometry") -> (appended path=w336:path)
            n259 = property class="VI"(reference=w331, error in=w330, "Front Panel Window:Open"=TRUE) -> (reference out=w328:refnum<vi>, error out=w329:errorcluster)
            n260 = Build Path(base path=w336, name or relative path=w327) -> (appended path=w334:path)
            n261 = Close Reference(reference=w328, error in (no error)=w329) -> (error out=w326:errorcluster)
            n262 = Unbundle By Name(w326) -> ("status"=w335:bool)
            n263 = case shown="True" w335 {
              tunnel: w334 -> [_ w338]
              tunnel: w326 -> [_ _]
              frame False {
              }
              frame True {
                n264 = stacked-sequence {
                  seq-local: [w344 _] -> [_ w351]
                  tunnel: w338 -> [_ w352]
                  frame #0 {
                    n265 = call "Setup_Filepath.vi"("Setup File Type"=Setup_Filetype."Calibration Setups", "Filename in"="Current_Setup.xls") -> ("Filename Out"=w339:path)  [unwired: 1 out]
                    n266 = call "Read_File_Simple.vi"("Filename"=w339) -> ("string"=w348:string)  [unwired: 2 in, 7 out]
                    n267 = Format Into String(format string="Calibration Setup File   %s", w339) -> (resulting string=w342:string)  [unwired: 2 in, 1 out]
                    n268 = call "Get_string_subset.vi"("String Name"=w342, "String to split"=w348, "File Label"="Raw data header") -> ("Output string"=w346:string)  [unwired: 1 in, 1 out]
                    n269 = call "Get_Characters_from_string.vi"("Input string"=w346, "Variable name"="Calib filename") -> ("Value"=w345:string)  [unwired: 1 in, 1 out]
                    n270 = call "String_to_Pathname.vi"("Input String"=w345) -> ("path"=w344:path)
                  }
                  frame #1 {
                    n271 = call "Does_file_exist_(simple).vi"("Pathname"=w351) -> ("exists?"=w350:bool)
                    n272 = case shown="True" w350 {
                      tunnel: w352 -> [w353 w368]
                      tunnel: w351 -> [_ w362]
                      frame False {
                        n273 = call "Open_Close_Front_Panel.ph.vi"("Front Panel Window:Open"=TRUE, "VI path"=w353) -> ()  [unwired: 2 out]
                      }
                      frame True {
                        w360 = TRUE ("Front Panel Window:Open")
                        n274 = Open VI Reference(type specifier VI Refnum (for type only)=refnum<vi> refnum, vi path=w368) -> (vi reference=w366:refnum<vi>, error out=w361:errorcluster)  [unwired: 1 in, 3 out]
                        n275 = property class="VI Interface Type 6"(reference=w366, error in=w361, "Front Panel Window:Open"=w360, "Front Panel Window:Auto Center (Deprecated)"=w360) -> (reference out=w365:refnum<vi>, error out=w364:errorcluster)
                        n276 = call-by-ref "?"(reference=w365, error in=w364, "Mode"=Calib_mode."Setup Front Panel", "Calib file"=w362) -> (reference out=w358:refnum<vi>, error out=w357:errorcluster)  [unwired: 15 in, 3 out]
                        n277 = property class="VI Interface Type 6"(reference=w358, error in=w357, "Front Panel Window:Auto Center (Deprecated)"=FALSE ("Front Panel Window:Auto Center")) -> (reference out=w356:refnum<vi>, error out=w355:errorcluster)
                        n278 = Close Reference(reference=w356, error in (no error)=w355) -> ()  [unwired: 1 out]
                      }
                    }
                  }
                }
              }
            }
            n279 = event-data() -> ()  [unwired: 1 in, 5 out]
          }
          event "stop": Mouse Down? {
            n280 = event-data() -> ()  [unwired: 5 out]
            n281 = flat-sequence {
              frame #0 {
                n282 = global write "Dynamic_call_global.ph.vi" "EnFlo Hub running?"(FALSE ("EnFlo Hub running?")) -> ()
              }
              frame #1 {
                n283 = Stop(stop? (T)=TRUE) -> ()
              }
            }
            n284 = event-data() -> ()  [unwired: 1 in, 4 out]
          }
          event "Rig_Control": Value Change {
            n285 = event-data() -> ("OldVal"=w372:cluster{"Ch Name":string, "Boolean":bool}[], "NewVal"=w371:cluster{"Ch Name":string, "Boolean":bool}[])  [unwired: 5 out]
            n286 = for {
              tunnel: w372 -> [w378] mode=indexing
              tunnel: w371 -> [w377] mode=indexing
              n287 = Unbundle By Name(w378) -> ("Ch Name"=w375:string, "Boolean"=w376:bool)
              n288 = Unbundle By Name(w377) -> ("Boolean"=w374:bool)  [unwired: 1 out]
              n289 = Not Equal?(x=w376, y=w374) -> (x != y?=w373:bool)
              n290 = case shown="True" w373 {
                tunnel: w375 -> [_ w380]
                tunnel: w374 -> [_ w387]
                frame False {
                }
                frame True {
                  n291 = Select(t="TRUE", s=w387, f="FALSE") -> (s? t:f=w379:string)
                  n292 = Select(t=1.0, s=w387, f=0.0) -> (s? t:f=w386:dbl)
                  n293 = Format Into String(format string="Are you sure you want to make %s %s?", w380, w379) -> (resulting string=w389:string)  [unwired: 2 in, 1 out]
                  n294 = Format Into String(format string="Make  %s  %s", w380, w379) -> (resulting string=w381:string)  [unwired: 2 in, 1 out]
                  n295 = Two Button Dialog(message=w389, 1:w381, 2:"Cancel" ("T button name (\"OK\")")) -> (T button?=w383:bool)
                  n296 = case shown="False" w383 {
                    tunnel: w380 -> [w394 _]
                    tunnel: w386 -> [w393 _]
                    frame False {
                      n297 = Build Array(w393) -> (w396:dbl[])
                      n298 = Build Array(w394) -> (w395:string[])
                      n299 = call "ASYNC_Adam_client.vi"("Values"=w396, "Channel Names"=w395) -> ()  [unwired: 2 out]
                    }
                    frame True {
                    }
                  }
                }
              }
            }
          }
          event Mouse Down? {
            w403 = TRUE  # Show Panel
            n300 = event-data() -> ()  [unwired: 5 out]
            n301 = global read "Constants_global.vi" "EnFlo SW Folder"() -> (w397:path)
            n302 = Build Path(base path=w397, name or relative path=path "Anemometry/Anemometry Sub Vis/LDA/Enter_LDA_Setup.vi") -> (appended path=w401:path)
            n303 = Open VI Reference(type specifier VI Refnum (for type only)=refnum<vi> refnum, vi path=w401) -> (vi reference=w404:refnum<vi>, error out=w405:errorcluster)  [unwired: 1 in, 3 out]
            n304 = call-by-ref "?"(reference=w404, error in=w405, "Show Panel"=w403) -> (reference out=w399:refnum<vi>, error out=w400:errorcluster)
            n305 = Close Reference(reference=w399, error in (no error)=w400) -> ()  [unwired: 1 out]
            n306 = event-data() -> ()  [unwired: 1 in, 4 out]
          }
        }
      }
    }
    "Numeric" <- w8
  }
  n307 = while {
    shift-left: _ -> [w410]
    shift-right: [w411] -> _
    shift-left: "Initialise" -> [w409]
    shift-right: [w412] -> _
    tunnel: "ADAM_Chs_to_Enable.txt" ("name or relative path") -> [w407]
    tunnel: "ADAM_Chs_to_View.txt" ("name or relative path") -> [w406]
    i -> [w408]
    stop <- TRUE continue-if-true
    n308 = case shown="\"Initialise\"" w409 {
      tunnel: ["End" "Initialise" "Wait for call remote sub vi occurrence" "Check type of VI to launch" w485 "Wait until remote sub vi is opened" "Update opened vis array" "Update opened vis array" "Update opened vis array" "Wait until remote sub vi is opened" "Wait for call remote sub vi occurrence"] -> w412
      tunnel: [w414 w429 w434 errorcluster {"status"=FALSE, "code"=0, "source"=""} ("error out") w481 w496 w526 w543 w558 w598 w618] -> w411
      tunnel: w410 -> [w414 w429 w434 _ w481 w496 _ _ _ w598 w618]
      tunnel: w409 -> [w416 _ _ _ _ _ _ _ _ _ _]
      tunnel: w408 -> [_ _ _ _ _ _ _ _ _ _ _]
      tunnel: w407 -> [_ _ w431 _ _ _ _ _ _ _ _]
      tunnel: w406 -> [_ _ w430 _ _ _ _ _ _ _ _]
      frame "No match", Default {
        n309 = Current VI's Path() -> (path=w417:path)
        n310 = Format Into String(format string="The Case\"%s\" was not Matched\nin VI named\n'%s\"" ("Format String"), w416, w417) -> (resulting string=w420:string)  [unwired: 2 in, 1 out]
        n311 = One Button Dialog(message=w420, button name ("OK")="STOP") -> (true=w418:bool)
        n312 = Stop(stop? (T)=w418) -> ()
      }
      frame "Never run" {
        # "These globals are here to make sure they stay in momory\nafter \"Preference Panel\" has finished running"
        n313 = call "Email_With_Log.vi"() -> ()  [unwired: 4 in, 3 out]
        n314 = call "Remember_value.vi"() -> ()  [unwired: 3 in, 1 out]
        n315 = call "Read_Write_Local_table.vi"() -> ()  [unwired: 3 in, 3 out]
        n316 = call "Overhead_Factor.vi"() -> ()  [unwired: 4 in, 1 out]
        n317 = global read "Trav_pos_global.vi" "Dummy Measurement?"() -> (→"Dummy Measurement":bool)
        n318 = global read "PWAtasksGLOBAL.vi" "Analogue Dev Name"() -> (→"Analogue Dev Name":string)
        n319 = global read "Dynamic_call_global.ph.vi" "Ready to take data?"() -> (→"Ready to take data?":T1)
        n320 = global read "Qnet_Globals.vi" "Local Site Root"() -> (→"Local Site Root":path)
        n321 = global read "Constants_global.vi" "All_Users"() -> (→"All Users":path)
        n322 = global read "Preference_global.vi" "Rig Setup"() -> (→"Rig Name":string)
      }
      frame "Initialise" {
        n323 = stacked-sequence {
          tunnel: w431 -> [_ _ _ _ w473]
          tunnel: w430 -> [_ _ _ _ w469]
          frame #0 {
            n324 = Generate Occurrence() -> (w456:refnum<k4>)
            n325 = global write "Dynamic_call_global.ph.vi" "Call Remote Subvi"(w456) -> ()
            n326 = Generate Occurrence() -> (w455:refnum<k4>)
            n327 = global write "Dynamic_call_global.ph.vi" "Remote Subvi Opened"(w455) -> ()
            n328 = Initialize Array("", 0) -> (w453:string[])
            n329 = global write "Dynamic_call_global.ph.vi" "Opened VIs"(w453) -> ()
            n330 = global write "Email_transfer_global.vi" "Busy?"(FALSE ("Busy?")) -> ()
            n331 = Current VI's Path() -> (path=w445:path)
            n332 = Strip Path(path=w445) -> (stripped path=w443:path)  [unwired: 1 out]
            n333 = Build Path(base path=w443, name or relative path="Utilities") -> (appended path=w441:path)
            n334 = Build Path(base path=w441, name or relative path="Preference_Panel.vi") -> (appended path=w440:path)
            n335 = Get Date/Time In Seconds() -> (seconds since 1Jan1904=w451:timestamp)
            n336 = To Double Precision Float(number=w451) -> (double precision float=w450:dbl)
            n337 = Open VI Reference(type specifier VI Refnum (for type only)=refnum<vi> refnum, vi path=w440) -> (vi reference=w446:refnum<vi>, error out=w447:errorcluster)  [unwired: 1 in, 3 out]
            n338 = Generate Occurrence() -> (w436:refnum<k4>)
            n339 = global write "Meas_global.vi" "Start Time of experiment"(w450) -> ()
            n340 = global write "Meas_global.vi" "Post Process"(Post_Process."Post Process Raw Data File" ("Post Process")) -> ()
            n341 = call-by-ref "?"(reference=w446, error in=w447, "Mode"=Preference_Mode."Load Preferences from file") -> (reference out=w448:refnum<vi>, error out=w449:errorcluster)
            n342 = global write "Dynamic_call_global.ph.vi" "Take data"(w436) -> ()
            n343 = Close Reference(reference=w448, error in (no error)=w449) -> ()  [unwired: 1 out]
          }
          frame #1 {
            w457 = TRUE  # OK
            n344 = call "Get_users_email_addresses.vi"("OK"=w457) -> ()  [unwired: 5 out]
          }
          frame #2 {
            n345 = Current VI's Path() -> (path=w466:path)
            n346 = Open VI Reference(vi path=w466) -> (vi reference=w465:refnum<vi>, error out=w464:errorcluster)  [unwired: 1 in, 4 out]
            n347 = call "Last_modified_date.vi"("Update Now"=TRUE) -> ("Programs last revision time"=w459:u32)  [unwired: 1 out]
            n348 = property class="VI"(reference=w465, error in=w464, "Front Panel Window:Open"=TRUE, "Front Panel Window:Is Frontmost"=FALSE) -> (reference out=w463:refnum<vi>, error out=w462:errorcluster)
            n349 = global write "Meas_global.vi" "Prog's last revision date"(w459) -> ()
            n350 = Close Reference(reference=w463, error in (no error)=w462) -> ()  [unwired: 1 out]
          }
          frame #3 {
            n351 = global write "Dynamic_call_global.ph.vi" "EnFlo Hub running?"(TRUE ("EnFlo Hub running?")) -> ()
          }
          frame #4 {
            n352 = global read "Constants_global.vi" "All_Users"() -> (w470:path)
            n353 = Build Path(base path=w470, name or relative path=w469) -> (appended path=w472:path)
            n354 = Build Path(base path=w470, name or relative path=w473) -> (appended path=w475:path)
            n355 = call "Read_File_Simple.vi"("Filename"=w472) -> ("string"=w471:string)  [unwired: 2 in, 7 out]
            n356 = call "Read_File_Simple.vi"("Filename"=w475) -> ("string"=w476:string)  [unwired: 2 in, 7 out]
            n357 = call "Get_array_values_fr_String.vi"("String Value"=w471) -> ("String array"=→"List of ADAM channels to view":string[])  [unwired: 1 out]
            n358 = call "Get_array_values_fr_String.vi"("String Value"=w476) -> ("String array"=→"List of ADAM control channels":string[])  [unwired: 1 out]
          }
        }
        "Iterations" <- 0 ("Iterations")
      }
      frame "Wait for call remote sub vi occurrence" {
        n359 = global read "Dynamic_call_global.ph.vi" "Call Remote Subvi"() -> (w479:refnum<k4>)
        n360 = Wait on Occurrence(2:w479) -> ()  [unwired: 3 out]
      }
      frame "Check type of VI to launch" {
        n361 = global read "Dynamic_call_global.ph.vi" "VI name to launch"() -> (w483:string)
        n362 = Match Pattern(string=w483, regular expression=";") -> (before substring=w480:string, after substring=w482:string)  [unwired: 3 out]
        n363 = case shown="\"Open LDA PWA & An\"" w480 {
          tunnel: ["Open vi" "Open application reference" "Open Analogue input server" w493] -> w485
          tunnel: [w488 w490 w492 w494] -> w484
          tunnel: w483 -> [w488 _ _ _]
          tunnel: w482 -> [_ w490 w492 w494]
          tunnel: w480 -> [_ _ _ w493]
          frame "Other", Default {
          }
          frame "Open Application Reference" {
          }
          frame "Open Analogue Input VI" {
          }
          frame "Open LDA PWA & An" {
          }
        }
        "VI Name" <- w484
      }
      frame "Open application reference" {
        n364 = local read "VI Name"() -> (w497:string)
        n365 = Match Pattern(string=w497, regular expression=";") -> (before substring=w505:string, after substring=w506:string)  [unwired: 3 out]
        n366 = Decimal String To Number(string=w506) -> (number=w507:i32)  [unwired: 3 out]
        n367 = To Unsigned Long Integer(number=w507) -> (unsigned 32bit integer=w504:u32)
        n368 = call "App_Ref_Global.vi"("Mode"=App_Global."Read Global") -> ("Output Array"=w503:T49[])  [unwired: 1 in, 1 out]
        n369 = Open Application Reference(10:w504, 11:w505) -> (0:w498:errorcluster, 3:w502:refnum<vi>)  [unwired: 1 in, 1 out]
        n370 = for {
          tunnel: w503 -> [w509] mode=indexing
          tunnel: w497 -> [w513]
          tunnel: w502 -> [w511]
          tunnel: [w510] -> w501 mode=indexing
          n371 = Unbundle By Name(w509) -> ("Server IP & Port No"=w514:string)
          n372 = Equal?(x=w514, y=w513) -> (x = y?=w512:bool)
          n373 = case shown="False" w512 {
            tunnel: w511 -> [_ w518]
            tunnel: [w515 w517] -> w510
            tunnel: w509 -> [w515 w516]
            frame False {
            }
            frame True {
              n374 = Bundle By Name(cluster=w516, "Application reference"=w518) -> (w517:T49)
            }
          }
        }
        n375 = global write "Dynamic_call_global.ph.vi" "Error Cluster"(w498) -> ()
        n376 = call "App_Ref_Global.vi"("Input Array"=w501, "Mode"=App_Global."Write to Global") -> ()  [unwired: 2 out]
      }
      frame "Open Analogue input server" {
        n377 = local read "VI Name"() -> (w523:string)
        n378 = call "Get_link_info.vi"("VI Name"=w523) -> ("Path name"=w520:path, "Application reference"=w521:refnum<vi>, "Local Call?"=w522:bool)  [unwired: 1 out]
        n379 = global read "Dynamic_call_global.ph.vi" "Analogue Input"() -> (w525:refnum<vi>)
        n380 = case shown="True" w522 {
          tunnel: w525 -> [w531 w535]
          tunnel: [w527 w534] -> w524
          tunnel: [w530 w533] -> w526
          tunnel: w523 -> [w529 _]
          tunnel: w521 -> [w528 _]
          tunnel: w520 -> [_ w532]
          frame False {
            n381 = Open VI Reference(type specifier VI Refnum (for type only)=w531, application reference (local)=w528, vi path=w529) -> (vi reference=w527:refnum<vi>, error out=w530:errorcluster)  [unwired: 1 in, 2 out]
          }
          frame True {
            n382 = Open VI Reference(type specifier VI Refnum (for type only)=w535, vi path=w532) -> (vi reference=w534:refnum<vi>, error out=w533:errorcluster)  [unwired: 1 in, 3 out]
          }
        }
        n383 = global write "Dynamic_call_global.ph.vi" "Analogue Input"(w524) -> ()
      }
      frame "Open LDA PWA & An" {
        n384 = local read "VI Name"() -> (w540:string)
        n385 = call "Get_link_info.vi"("VI Name"=w540) -> ("Path name"=w537:path, "Application reference"=w538:refnum<vi>, "Local Call?"=w539:bool)  [unwired: 1 out]
        n386 = global read "Dynamic_call_global.ph.vi" "Take LDA PWA & An"() -> (w542:refnum<vi>)
        n387 = case shown="True" w539 {
          tunnel: w542 -> [w548 w552]
          tunnel: [w544 w551] -> w541
          tunnel: [w547 w550] -> w543
          tunnel: w540 -> [w546 _]
          tunnel: w538 -> [w545 _]
          tunnel: w537 -> [_ w549]
          frame False {
            n388 = Open VI Reference(type specifier VI Refnum (for type only)=w548, application reference (local)=w545, vi path=w546) -> (vi reference=w544:refnum<vi>, error out=w547:errorcluster)  [unwired: 1 in, 2 out]
          }
          frame True {
            n389 = Open VI Reference(type specifier VI Refnum (for type only)=w552, vi path=w549) -> (vi reference=w551:refnum<vi>, error out=w550:errorcluster)  [unwired: 1 in, 3 out]
          }
        }
        n390 = global write "Dynamic_call_global.ph.vi" "Take LDA PWA & An"(w541) -> ()
      }
      frame "Open vi" {
        n391 = local read "VI Name"() -> (w557:string)
        n392 = call "Get_link_info.vi"("VI Name"=w557) -> ("Path name"=w556:path, "Application reference"=w555:refnum<vi>, "Local Call?"=w554:bool)  [unwired: 1 out]
        n393 = case shown="\"No Match\", Default" w557 {
          tunnel: [w559 w568 w580] -> w558
          tunnel: w557 -> [w564 w567 w584]
          tunnel: w556 -> [_ _ w581]
          tunnel: w555 -> [_ w566 w583]
          tunnel: w554 -> [_ w565 w582]
          frame "No Match", Default {
            n394 = Format Into String(format string="VI named \"%s\" Not matched" ("Format String"), w564) -> (resulting string=w561:string)  [unwired: 2 in, 1 out]
            n395 = Bundle By Name(cluster=errorcluster {"status"=FALSE, "code"=0, "source"=""} ("error out"), "source"=w561, "status"=TRUE ("Bundle Element")) -> (w559:errorcluster)
          }
          frame "Program_Active_server.vi" {
            n396 = global read "Dynamic_call_global.ph.vi" "Program Active server"() -> (w570:refnum<vi>)
            n397 = case shown="True" w565 {
              tunnel: w570 -> [w575 w579]
              tunnel: [w574 w578] -> w569
              tunnel: [w573 w577] -> w568
              tunnel: w567 -> [w572 w576]
              tunnel: w566 -> [w571 _]
              frame False {
                n398 = Open VI Reference(type specifier VI Refnum (for type only)=w575, application reference (local)=w571, vi path=w572) -> (vi reference=w574:refnum<vi>, error out=w573:errorcluster)  [unwired: 1 in, 2 out]
              }
              frame True {
                n399 = Open VI Reference(type specifier VI Refnum (for type only)=w579, vi path=w576) -> (vi reference=w578:refnum<vi>, error out=w577:errorcluster)  [unwired: 1 in, 3 out]
              }
            }
            n400 = global write "Dynamic_call_global.ph.vi" "Program Active server"(w569) -> ()
          }
          frame "GPIB_Server.vi" {
            n401 = global read "Dynamic_call_global.ph.vi" "GPIB_Server.vi"() -> (w586:refnum<vi>)
            n402 = case shown="False" w582 {
              tunnel: w586 -> [w591 w595]
              tunnel: [w590 w594] -> w585
              tunnel: [w589 w593] -> w580
              tunnel: w584 -> [w587 _]
              tunnel: w583 -> [w588 _]
              tunnel: w581 -> [_ w592]
              frame False {
                n403 = Open VI Reference(type specifier VI Refnum (for type only)=w591, application reference (local)=w588, vi path=w587) -> (vi reference=w590:refnum<vi>, error out=w589:errorcluster)  [unwired: 1 in, 2 out]
              }
              frame True {
                n404 = Open VI Reference(type specifier VI Refnum (for type only)=w595, vi path=w592) -> (vi reference=w594:refnum<vi>, error out=w593:errorcluster)  [unwired: 1 in, 3 out]
              }
            }
            n405 = global write "Dynamic_call_global.ph.vi" "GPIB_Server.vi"(w585) -> ()
          }
        }
      }
      frame "Update opened vis array" {
        w600 = TRUE  # Dialog Box
        n406 = local read "VI Name"() -> (w599:string)
        n407 = Unbundle By Name(w598) -> ("status"=w603:bool, "source"=w601:string)
        n408 = case shown="True" w603 {
          tunnel: w598 -> [w605 w614]
          tunnel: [w605 w613] -> w602
          tunnel: w599 -> [w606 w609]
          tunnel: w601 -> [_ w612]
          frame False {
            n409 = To Upper Case(1:w606) -> (0:w604:string)
            n410 = global read "Dynamic_call_global.ph.vi" "Opened VIs"() -> (w607:string[])
            n411 = Build Array (concatenate)(w607, w604) -> (w608:string[])
            n412 = global write "Dynamic_call_global.ph.vi" "Opened VIs"(w608) -> ()
          }
          frame True {
            n413 = Concatenate Strings(w609, " " ("Substring"), w612) -> (w610:string)
            n414 = Bundle By Name(cluster=w614, "source"=w610) -> (w613:errorcluster)
          }
        }
        n415 = call "EnFlo_Error_Handler.vi"("error in (no error)"=w602, "Error Type"="Dynamic Call", "Dialog Box (T)"=w600) -> ()  [unwired: 3 out]
      }
      frame "Wait until remote sub vi is opened" {
        n416 = global read "Dynamic_call_global.ph.vi" "Remote Subvi Opened"() -> (w619:refnum<k4>)
        n417 = local read "Iterations"() -> (w617:i32)
        n418 = Increment(x=w617) -> (x+1=w616:i32)
        n419 = local write "Iterations"(w616) -> ()
        n420 = Set Occurrence(w619) -> ()
      }
    }
  }
  n421 = while {
    stop <- FALSE stop-if-true
    n422 = global read "Dynamic_call_global.ph.vi" "EnFlo Hub running?"() -> (w621:bool)
    n423 = Equal?(x="Tab Control", y=T2."Adam Table" ("Tab Control")) -> (x = y?=w622:bool)
    n424 = And(x=w622, y=w621) -> (x .and. y?=w620:bool)
    n425 = case shown="True" w620 {
      frame True {
        n426 = local read "List of ADAM channels to view"() -> (w633:string[])
        n427 = local read "List of ADAM control channels"() -> (w636:string[])
        n428 = Build Array (concatenate)(w636, w633) -> (w635:string[])
        n429 = call "Get_Current_Scan_client.vi"("ADAM Ch Names"=w635) -> ("Ch Description Array"=w630:T50[], "Numerical Values"=w634:dbl[])  [unwired: 2 out]
        n430 = Array Size(array=w636) -> (size(s)=w631:i32)
        n431 = Array Subset(array=w630, index=w631) -> (w629:T50[])  [unwired: 1 in]
        n432 = Array Subset(array=w634, index=w631) -> (w628:dbl[])  [unwired: 1 in]
        n433 = for {
          tunnel: w629 -> [w643] mode=indexing
          tunnel: [w642] -> w627 mode=indexing
          tunnel: cluster{"Ch Name":string, "Numeric":dbl} {"Ch Name"="", "Numeric"=0.0} ("Cluster") -> [w641]
          tunnel: w628 -> [w639] mode=indexing
          n434 = Unbundle By Name(w643) -> ("Ch Name"=w640:string)
          n435 = Bundle By Name(cluster=w641, "Ch Name"=w640, "Numeric"=w639) -> (w642:cluster{"Ch Name":string, "Numeric":dbl})
        }
        "Current Values" <- w627
        n436 = for {
          N: w631 -> [_]
          tunnel: cluster{"Ch Name":string, "Boolean":bool} {"Ch Name"="", "Boolean"=FALSE} ("Cluster") -> [w650]
          tunnel: w630 -> [w649] mode=indexing
          tunnel: w634 -> [w647] mode=indexing
          tunnel: [w644] -> w637 mode=indexing
          n437 = Unbundle By Name(w649) -> ("Ch Name"=w648:string)
          n438 = Greater?(x=w647, y=0.5) -> (0:w645:bool)
          n439 = Bundle By Name(cluster=w650, "Ch Name"=w648, "Boolean"=w645) -> (w644:cluster{"Ch Name":string, "Boolean":bool})
        }
        n440 = local write "Rig_Control"(w637) -> ()
      }
      frame False {
      }
    }
    n441 = Wait (ms)(milliseconds to wait=u32 1000) -> ()  [unwired: 1 out]
  }
